vi "Worksheet Data to Measurement Definitions Dictionary.vi"(8 "error in (no error)":errorcluster, 10 "Worksheet Data":string[][](array[string]), 11 "NI Generic Parser in":refnum<class "NI Generic Parser.lvclass">) -> (0 "error out":errorcluster, 3 "NI Generic Parser out":refnum<class "NI Generic Parser.lvclass">)   [LabVIEW 2016, in "NI Generic Parser.lvlib" / "NI Generic Parser.lvclass"]
uses:
  NI Generic Parser.lvclass
  NI Generic Parser.lvclass/NI Generic Parser.ctl
  Plugins/Measurement Data.lvlibp/Controls/Measurement Description.ctl
  Plugins/Measurement Data.lvlibp/Controls/Measurement Position.ctl
  Plugins/String Database.lvlibp/String Database.lvclass
  Protected Methods/Read Measurement Description Dictionary.vi
  Protected Methods/Write Measurement Description Dictionary.vi
  Support/Step Sequence Database/Multi Step Database.lvclass
  Plugins/Measurement Data.lvlibp/Measurement Data.lvclass
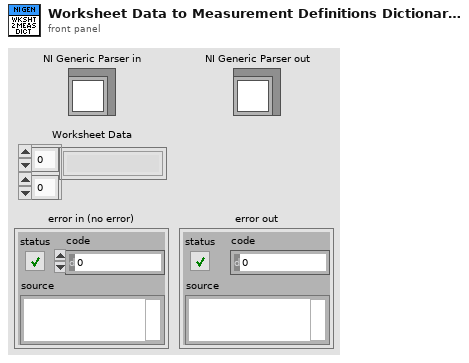
[diagram p1: front panel]
types:
  T1 = typedef "Measurement Data.lvlibp/Measurement Data.lvclass/Measurement Description.ctl" = cluster{"Measurement Sequence Position":T2, "Measurement Data":refnum<class "String Database.lvclass">, "Measurement Definition Entry":string}
  T2 = typedef "Measurement Data.lvlibp/Measurement Data.lvclass/Measurement Position.ctl" = enum16{"PreMeasurement", "MainMeasurement", "PostMeasurement"}
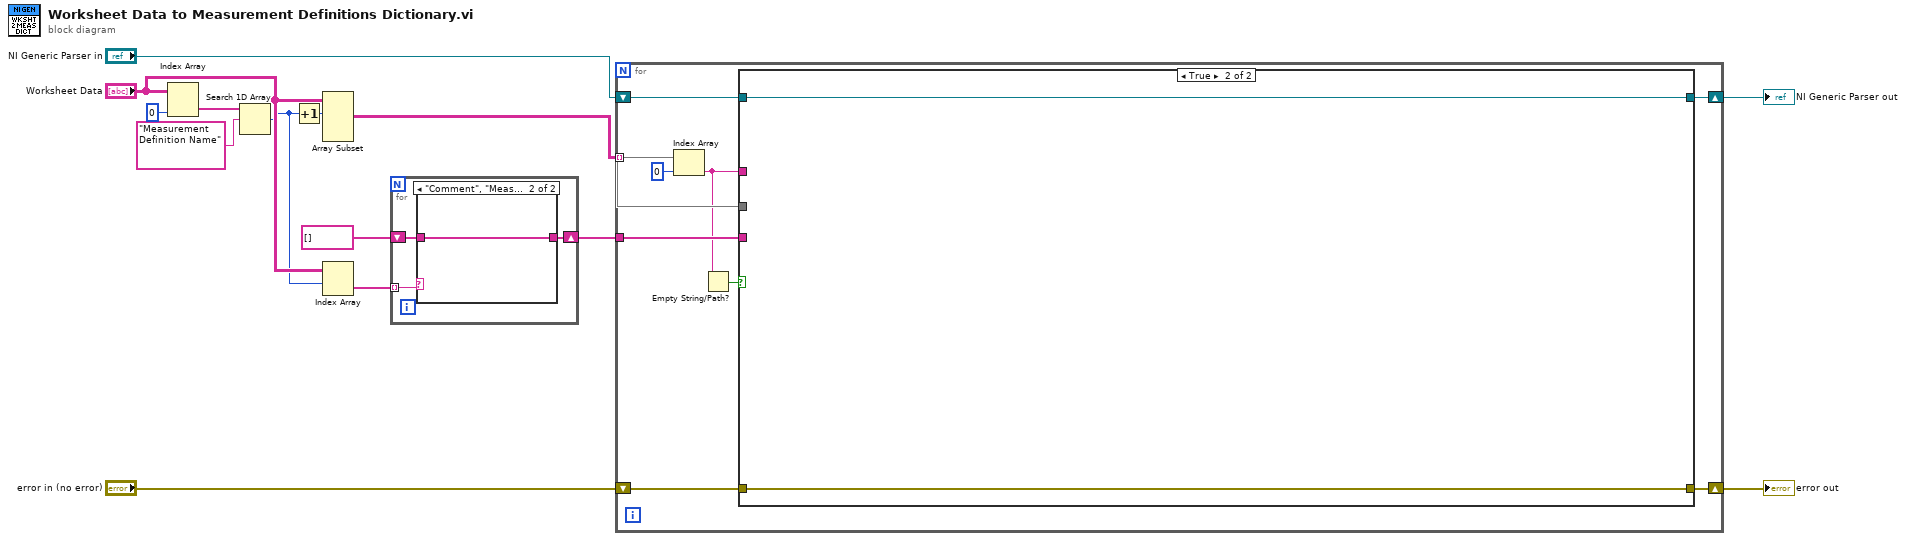
[diagram p0: block diagram]
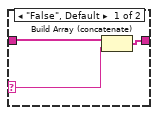
[diagram p2: hidden frame]
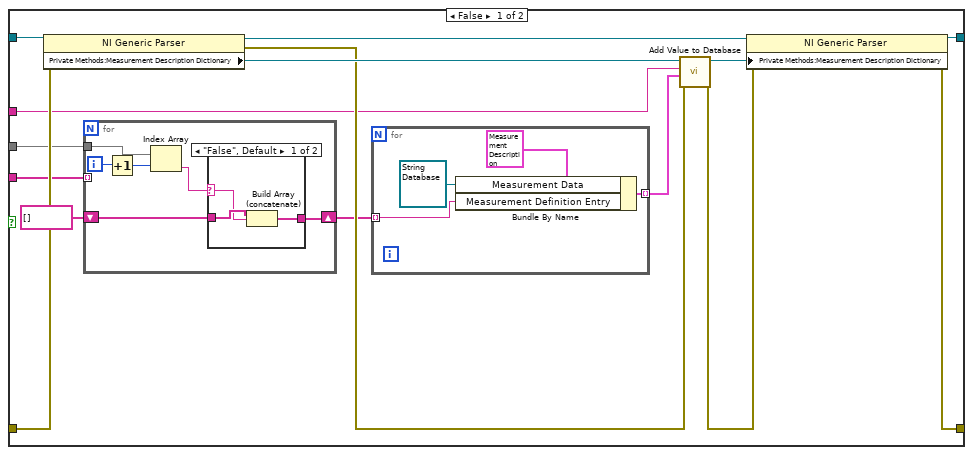
[diagram p3: hidden frame]
diagram:
  n1 = Index Array(array="Worksheet Data", index (col)=0 ("disabled index (col)")) -> (element=w9:string[])  [unwired: 1 in]
  n2 = Search 1D Array(1D array=w9, element="Measurement Definition Name") -> (index of element=w5:i32)  [unwired: 1 in]
  n3 = Increment(x=w5) -> (x+1=w1:i32)
  n4 = Array Subset(array="Worksheet Data", index (row)=w1) -> (w7:string[][])  [unwired: 3 in]
  n5 = Index Array(array="Worksheet Data", index (row)=w5) -> (element=w4:string[])  [unwired: 1 in]
  n6 = for {
    tunnel: w4 -> [w17] mode=indexing
    shift-right: [w15] -> w2
    shift-left: string[] [] -> [w16]
    n7 = case shown="\"Comment\", \"Measurement Definition Name\"" w17 {
      selector: w17 -> [w19 _]
      tunnel: w16 -> [w20 w21]
      tunnel: [w18 w21] -> w15
      frame "False", Default {
        n8 = Build Array (concatenate)(w20, w19) -> (w18:string[])
      }
      frame "Comment", "Measurement Definition Name" {
      }
    }
  }
  n9 = for {
    shift-right: [w28] -> w12
    shift-left: "NI Generic Parser in" -> [w30]
    tunnel: w7 -> [w24] mode=indexing
    shift-right: [w27] -> w14
    shift-left: "error in (no error)" -> [w29]
    tunnel: w2 -> [w25]
    n10 = Index Array(array=w24, index=0) -> (element=w22:string)
    n11 = Empty String/Path?(string/path=w22) -> (empty?=w23:bool)
    n12 = case shown="True" w23 {
      tunnel: w30 -> [w45 w61]
      tunnel: w29 -> [w44 w60]
      tunnel: [w41 w61] -> w28
      tunnel: [w38 w60] -> w27
      tunnel: w22 -> [w36 _]
      tunnel: w25 -> [w35 _]
      tunnel: w24 -> [w34 _]
      frame False {
        n13 = property class="NI Generic Parser"(reference=w45, error in=w44) -> (reference out=w40:refnum<class "NI Generic Parser.lvclass">, error out=w42:errorcluster, "Private Methods:Measurement Description Dictionary"=w43:refnum<class "Multi Step Database.lvclass">)
        n14 = for {
          tunnel: w35 -> [_] mode=indexing
          tunnel: w34 -> [w55]
          shift-right: [w50] -> w32
          shift-left: string[] [] -> [w51]
          i -> [w54]
          n15 = Increment(x=w54) -> (x+1=w53:i32)
          n16 = Index Array(array=w55, index=w53) -> (element=w52:string)
          n17 = case shown="\"False\", Default" w52 {
            selector: w52 -> [w57 _]
            tunnel: w51 -> [w58 w59]
            tunnel: [w56 w59] -> w50
            frame "False", Default {
              n18 = Build Array (concatenate)(w58, w57) -> (w56:string[])
            }
            frame "", "NA" {
            }
          }
        }
        n19 = for {
          tunnel: w32 -> [w47] mode=indexing
          tunnel: [w46] -> w31 mode=indexing
          n20 = Bundle By Name(cluster=T1 {"Measurement Sequence Position"=enum."PreMeasurement", "Measurement Data"=refnum, "Measurement Definition Entry"=""} ("Measurement Data"), "Measurement Data"=refnum<class "String Database.lvclass"> refnum, "Measurement Definition Entry"=w47) -> (w46:T1)
        }
        n21 = call "Add Value to Database.vi"("error in (no error)"=w42, "Array"=w31, "Measurement Name"=w36, "Multi Step Database in"=w43) -> ("error out"=w39:errorcluster, "Multi Step Database out"=w37:refnum<class "Multi Step Database.lvclass">)  [unwired: 6 in]
        n22 = property class="NI Generic Parser"(reference=w40, error in=w39, "Private Methods:Measurement Description Dictionary"=w37) -> (reference out=w41:refnum<class "NI Generic Parser.lvclass">, error out=w38:errorcluster)
      }
      frame True {
      }
    }
  }
  "error out" <- w14
  "NI Generic Parser out" <- w12
